vi "setData.vi"(8 "error in (no error)":errorcluster, 10 "Data":variant, 11 "Message in":refnum<class "Message.lvclass">) -> (0 "error out":errorcluster, 3 "Message out":refnum<class "Message.lvclass">)   [LabVIEW 2009, in "Message.lvclass"]
uses:
  Message.lvclass
  Message.lvclass/Message.ctl
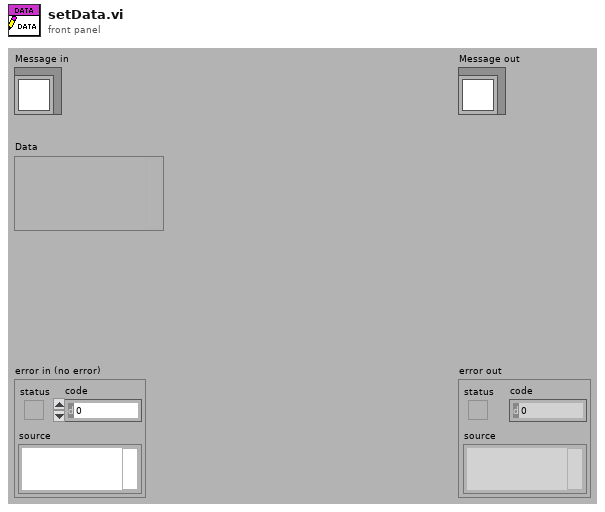
[diagram p1: front panel]
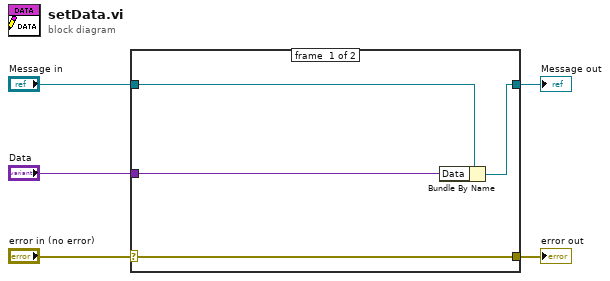
[diagram p0: block diagram]
diagram:
  n1 = case shown="No Error" "error in (no error)" {
    selector: "error in (no error)" -> [w9 w10]
    tunnel: [w9 w10] -> w4
    tunnel: [w7 w11] -> w2
    tunnel: "Message in" -> [w8 w11]
    tunnel: "Data" -> [w6 _]
    frame #0 {
      n2 = Bundle By Name(cluster=w8, "Data"=w6) -> (w7:refnum<class "Message.lvclass">)
    }
    frame #1 {
    }
  }
  "error out" <- w4
  "Message out" <- w2
